vi "formatStringElectrode.vi"(5 "Counter Electrode":T1(radio)=enum."Electrode 1", 6 "Reference Electrode":T1(radio)=enum."Electrode 1", 7 "Working Electrode":T1(radio)=enum."Electrode 1") -> (0 "Counter":u32, 1 "Active Reference":u32, 2 "Active Electrode":u32, 3 "output string":string)   [LabVIEW 2015]
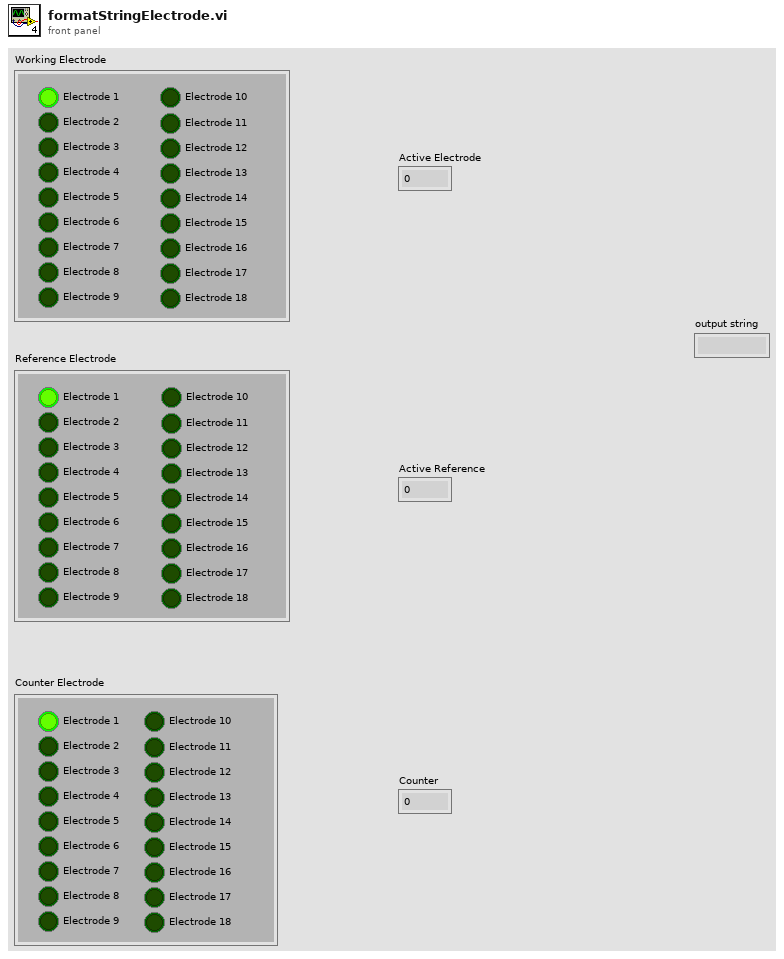
[diagram p1: front panel]
types:
  T1 = enum32{"No Selection", "Electrode 1", "Electrode 2", "Electrode 3", "Electrode 4", "Electrode 5", "Electrode 6", "Electrode 7", "Electrode 8", "Electrode 9", "Electrode 10", "Electrode 11", "Electrode 12", "Electrode 13", "Electrode 14", "Electrode 15", "Electrode 16", "Electrode 17", "Electrode 18"}
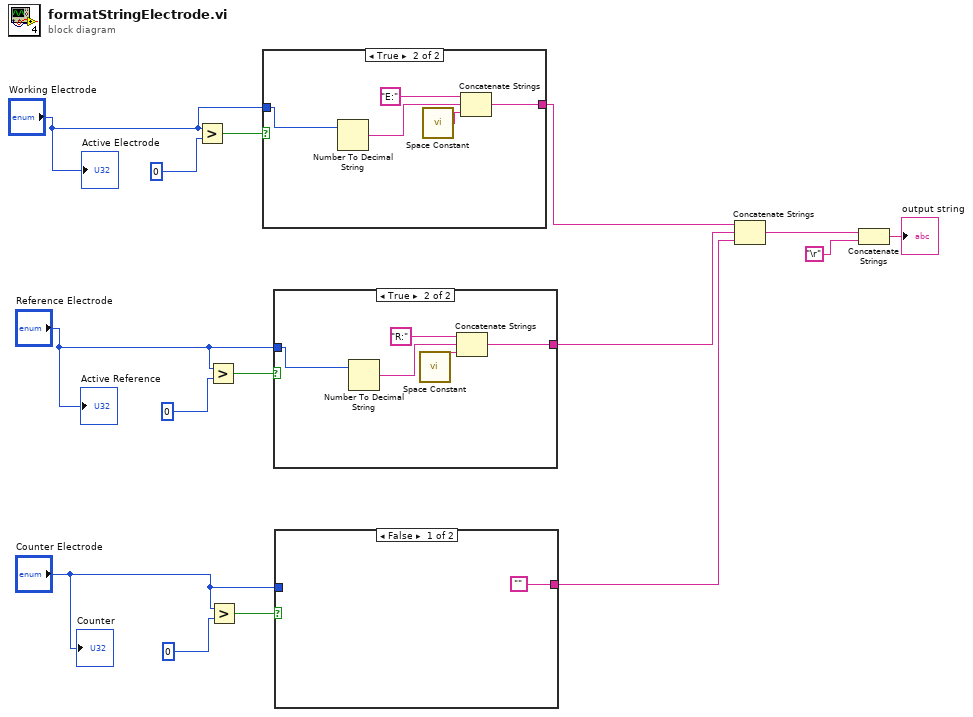
[diagram p0: block diagram]
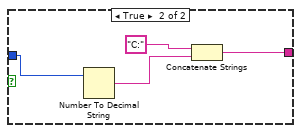
[diagram p2: hidden frame]
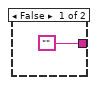
[diagram p3: hidden frame]
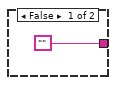
[diagram p4: hidden frame]
diagram:
  n1 = Greater?(x="Working Electrode", y=0) -> (0:w11:bool)
  n2 = Greater?(x="Reference Electrode", y=0) -> (0:w10:bool)
  n3 = Greater?(x="Counter Electrode", y=0) -> (0:w8:bool)
  n4 = case shown="True" w11 {
    tunnel: "Working Electrode" -> [_ w21]
    tunnel: ["" w18] -> w1
    frame False {
    }
    frame True {
      n5 = Number To Decimal String(number=w21) -> (decimal integer string=w20:string)  [unwired: 1 in]
      n6 = call <vilib>:"Space Constant.vi"() -> ("String"=w17:string)
      n7 = Concatenate Strings("E:" ("string"), w20, w17) -> (w18:string)
    }
  }
  n8 = case shown="True" w10 {
    tunnel: "Reference Electrode" -> [_ w27]
    tunnel: ["" w24] -> w2
    frame False {
    }
    frame True {
      n9 = Number To Decimal String(number=w27) -> (decimal integer string=w26:string)  [unwired: 1 in]
      n10 = call <vilib>:"Space Constant.vi"() -> ("String"=w23:string)
      n11 = Concatenate Strings("R:" ("string"), w26, w23) -> (w24:string)
    }
  }
  n12 = case shown="False" w8 {
    tunnel: "Counter Electrode" -> [_ w32]
    tunnel: ["" w29] -> w3
    frame False {
    }
    frame True {
      n13 = Number To Decimal String(number=w32) -> (decimal integer string=w31:string)  [unwired: 1 in]
      n14 = Concatenate Strings("C:" ("string"), w31) -> (w29:string)
    }
  }
  n15 = Concatenate Strings(w1, w2, w3) -> (w4:string)
  n16 = Concatenate Strings(w4, "\r") -> (→"output string":string)
  "Active Electrode" <- "Working Electrode"
  "Active Reference" <- "Reference Electrode"
  "Counter" <- "Counter Electrode"
